vi "Joystick Global 6740.vi"() -> ()   [LabVIEW 2019, in "Untitled Library 1.lvlib"]
uses:
  Untitled Library 1.lvlib
panel:
  in  "[F310] POVs":i16[](array[numeric])
  out "[F310] Right Joystick Button":bool
  out "[F310] .Y":bool
  out "[F310] .B":bool
  out "[F310] Start":bool
  out "[F310] .RB":bool
  out "[F310] Left Joystick Button":bool
  out "[F310] Back":bool
  out "[F310] .LB":bool
  out "[F310] .X":bool
  out "[F310] .A":bool
  in  "[F310] Axis":T1
  out "[F310] Buttons":T2
  in  "[F310] Right Y":dbl
  in  "[F310] Right X":dbl
  in  "[F310] Right Trigger":dbl
  in  "[F310] Left Trigger":dbl
  in  "[F310] Left Y":dbl
  in  "[F310] Left X":dbl
  in  "Right X3D POVs":i16[](array[numeric])
  out "Right 12":bool
  out "Right 11":bool
  out "Right 10":bool
  out "Right 9":bool
  out "Right 8":bool
  out "Right 7":bool
  out "Right 6":bool
  out "Right 5":bool
  out "Right 4":bool
  out "Right 3":bool
  out "Right 2":bool
  out "Right 1":bool
  in  "Right Joystick Slider":dbl
  in  "Right Joystick Y Axis":dbl
  in  "Right Joystick Z Axis":dbl
  in  "Right Joystick X Axis":dbl
  in  "Right X3D Joystick Axis":T3
  out "Right X3D Joystick Buttons":T4
  in  "[Xbox] POVs":i16[](array[numeric])
  in  "Left X3D POVs":i16[](array[numeric])
  out "Left 12":bool
  out "Left 11":bool
  out "Left 10":bool
  out "Left 9":bool
  out "Left 8":bool
  out "Left 7":bool
  out "Left 6":bool
  out "Left 5":bool
  out "Left 4":bool
  out "Left 3":bool
  out "Left 2":bool
  out "Left 1":bool
  in  "Left Joystick Slider":dbl
  in  "Left Joystick Y Axis":dbl
  in  "Left Joystick Z Axis":dbl
  in  "Left Joystick X Axis":dbl
  in  "Left X3D Joystick Axis":T3
  out "Left X3D Joystick Buttons":T4
  out "[Xbox] Right Joystick Button":bool
  out "[Xbox] .Y":bool
  out "[Xbox] .B":bool
  out "[Xbox] Start":bool
  out "[Xbox] .RB":bool
  out "[Xbox] Left Joystick Button":bool
  out "[Xbox] Back":bool
  out "[Xbox] .LB":bool
  out "[Xbox] .X":bool
  out "[Xbox] .A":bool
  in  "[Xbox] Axis":T1
  out "[Xbox] Buttons":T2
  in  "[Xbox] Right Y":dbl
  in  "[Xbox] Right X":dbl
  in  "[Xbox] Right Trigger":dbl
  in  "[Xbox] Left Trigger":dbl
  in  "[Xbox] Left Y":dbl
  in  "[Xbox] Left X":dbl
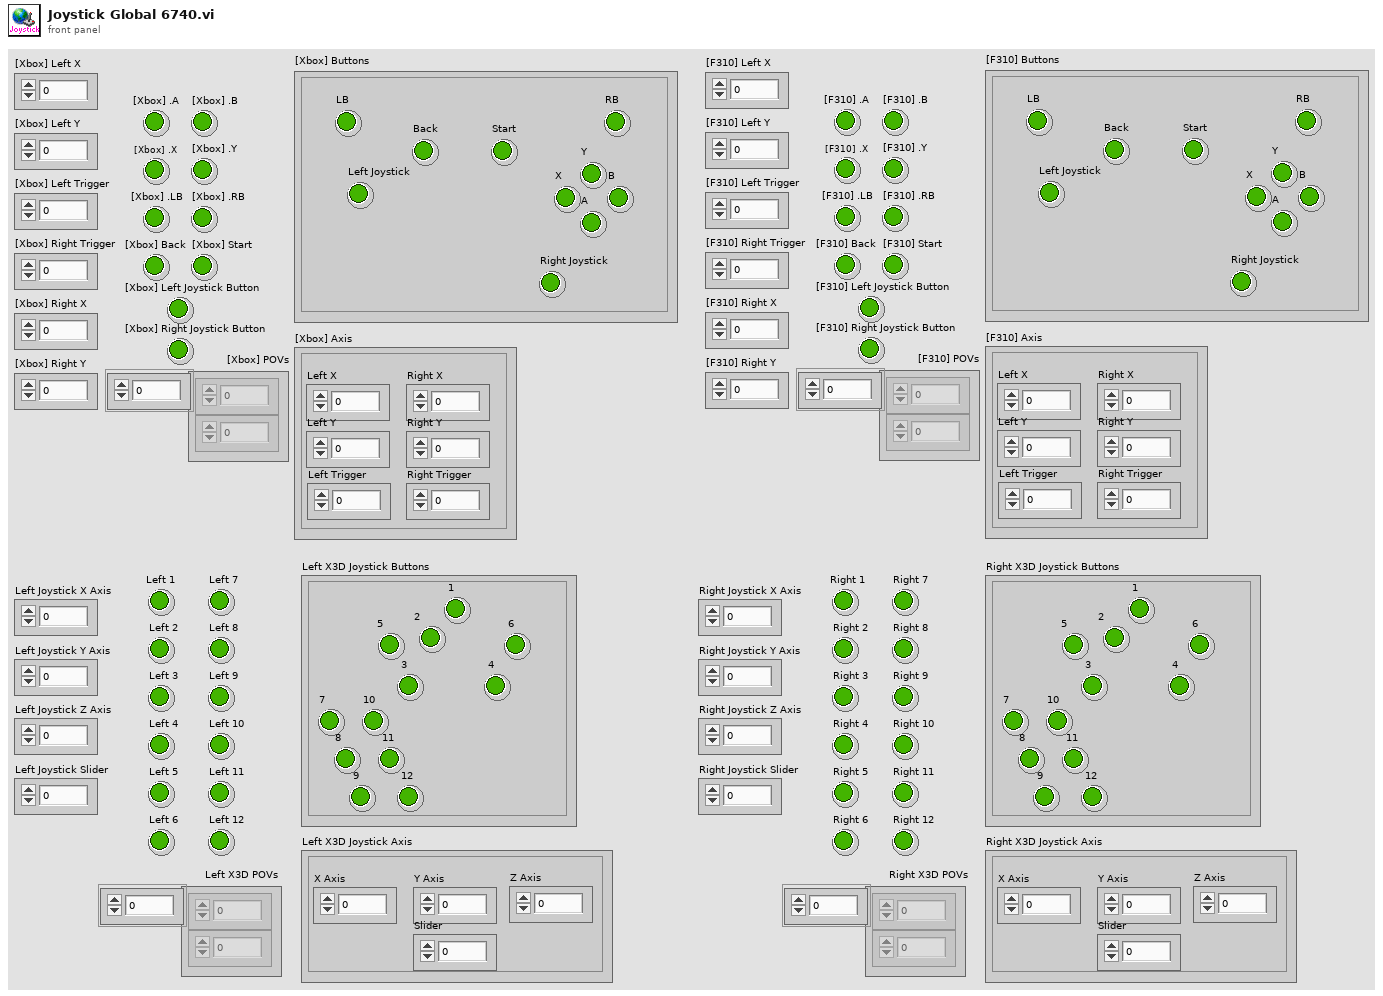
[diagram p1: front panel]
types:
  T1 = cluster{"Left X":dbl, "Left Y":dbl, "Left Trigger":dbl, "Right Trigger":dbl, "Right X":dbl, "Right Y":dbl}
  T2 = cluster{"A":bool, "B":bool, "X":bool, "Y":bool, "LB":bool, "RB":bool, "Back":bool, "Start":bool, "Left Joystick":bool, "Right Joystick":bool}
  T3 = cluster{"X Axis":dbl, "Y Axis":dbl, "Z Axis":dbl, "Slider":dbl}
  T4 = cluster{" 1":bool, " 2":bool, " 3":bool, " 5":bool, " 4":bool, " 6":bool, "7":bool, "8":bool, " 9":bool, "10":bool, " 11":bool, " 12":bool}
diagram:
